vi "Global Constants.vi"() -> ()   [LabVIEW 2014]
panel:
  in  "Tow-In BR":dbl
  in  "Tow-In BL":dbl
  in  "Tow-In FR":dbl
  in  "Tow-In FL":dbl
  in  "Rotational PID gains":T1={"proportional gain (Kc)"=0.01, "integral time (Ti, min)"=0.015, "derivative time (Td, min)"=0.0}
  in  "Header D":dbl=0.002 format="%_10g"
  in  "Header I":dbl=0.035 format="%_10g"
  in  "Header P":dbl=0.023 format="%_10g"
  in  "Robot Length":dbl=35.0
  in  "Robot Width":dbl=21.0
  in  "Resolver BR Low Voltage":dbl=0.196533
  in  "Resolver BR High Voltage":dbl=4.7229
  in  "Resolver BL Low Voltage":dbl=0.202637
  in  "Resolver BL High Voltage":dbl=4.70703
  in  "Resolver FR Low Voltage":dbl=0.203857
  in  "Resolver FR High Voltage":dbl=4.72778
  in  "Resolver FL Low Voltage":dbl=0.203857
  in  "Resolver FL High Voltage":dbl=4.7229
  in  "Example":dbl=1.0
  in  "Offset BR":dbl=-1.0
  in  "Offset BL":dbl=-1.0
  in  "Offset FR":dbl=-1.0
  in  "Offset FL":dbl=-1.0
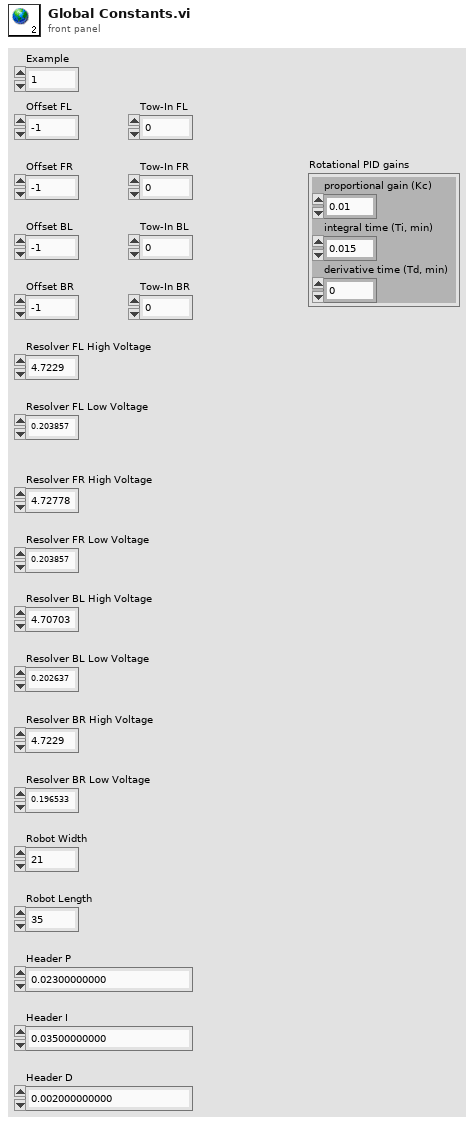
[diagram p1: front panel]
types:
  T1 = cluster{"proportional gain (Kc)":dbl, "integral time (Ti, min)":dbl, "derivative time (Td, min)":dbl}
diagram:
